vi "Reset_All_Positions.vi"(0 "Boolean":bool) -> ()   [LabVIEW 2013]
panel:
  out "P10":dbl[](array[numeric])
  out "P9":dbl[](array[numeric])
  out "P8":dbl[](array[numeric])
  out "P6":dbl[](array[numeric])
  out "P5":dbl[](array[numeric])
  out "P4":dbl[](array[numeric])
  out "P7":dbl[](array[numeric])
  out "P3":dbl[](array[numeric])
  out "P2":dbl[](array[numeric])
  out "P1":dbl[](array[numeric])
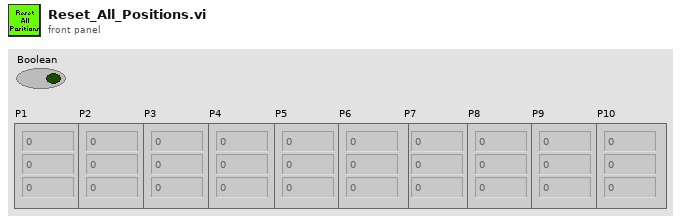
[diagram p1: front panel]
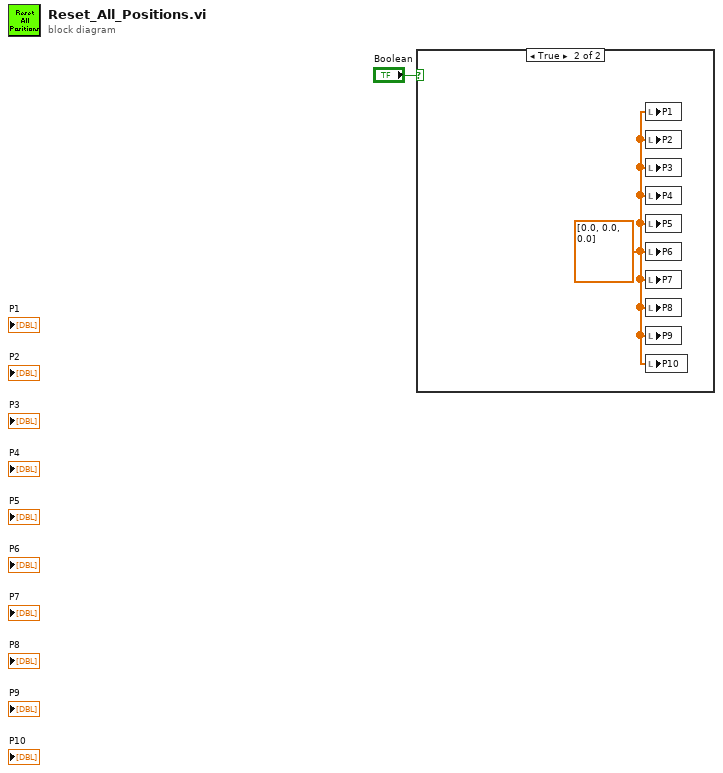
[diagram p0: block diagram]
diagram:
  n1 = case shown="True" "Boolean" {
    frame False {
    }
    frame True {
      w2 = dbl[] [0.0, 0.0, 0.0] ("P1")
      n2 = local write "P1"(w2) -> ()
      n3 = local write "P2"(w2) -> ()
      n4 = local write "P3"(w2) -> ()
      n5 = local write "P4"(w2) -> ()
      n6 = local write "P5"(w2) -> ()
      n7 = local write "P6"(w2) -> ()
      n8 = local write "P7"(w2) -> ()
      n9 = local write "P8"(w2) -> ()
      n10 = local write "P9"(w2) -> ()
      n11 = local write "P10"(w2) -> ()
    }
  }
